vi "Main.vi"(11 "Module Admin":refnum<class "Delacor_lib_QMH_Module Admin.lvclass">) -> ()   [LabVIEW 2021, in "Main HMI.lvlib"]
doc: "This template is based off of the Queued Message Handler design pattern and the Queued Message Handler project template that ships with LabVIEW.\n\nThe main difference is that the queue is private to this module and communication between modules is performed via Broadcast and Request events.\n\nRequest events are wrapped in public API methods and are handled in the Event Handling Loop (EHL) of this VI. Any module can register for Broadcast events sent by this module. The EHL generates messages based on user interface actions.\n\nThe Message Handling Loop (MHL) processes messages generated by the EHL, or by other messages. The messages are string values, so new messages can be added easily to the Message Cases case structure in the MHL. Each message cluster can also provide an optional value for Message Data, which is a variant that can be converted to whatever message-specific data is required.\n_____\nBased on DQMH Dev Tools: Project Template 7.1.2.1547."
uses:
  Main HMI.lvlib
  <vilib>/Delacor/Delacor QMH/Libraries/Module Admin_class/Delacor_lib_QMH_Module Admin.lvclass
  Module Data--cluster.ctl
  Get Measurement from UDP HL--cluster.ctl
  Stop Argument--cluster.ctl
  <vilib>/Delacor/Delacor QMH/Libraries/Message Queue_class/Delacor_lib_QMH_Message Queue.lvclass/Delacor_lib_QMH_Message Queue.ctl
  <vilib>/Delacor/Delacor QMH/Libraries/Module Admin_class/Delacor_lib_QMH_Module Admin.lvclass/Delacor_lib_QMH_Module Admin.ctl
  Open UDP Connection Argument--cluster.ctl
  <vilib>/Utility/miscctls.llb/LVPointTypeDef.ctl
  <vilib>/Delacor/Delacor QMH/Libraries/Message Queue_class/Delacor_lib_QMH_Enqueue Message (Single).vi
  <vilib>/Delacor/Delacor QMH/Libraries/Module Admin_class/Delacor_lib_QMH_Get External Launch.vi
  <vilib>/Delacor/Delacor QMH/Libraries/Message Queue_class/Delacor_lib_QMH_Message Queue.lvclass
  Host Interpreter/Host Interpreter.lvlib
panel:
  out "Connected":bool
  in  "Disconnect from Target":bool
  in  "Connect to Target":bool
  out "CPU 2 (%)":u8(slide) scale=0.0..100.0
  out "CPU 1 (%)":u8(slide) scale=0.0..100.0
  out "Memory ROM Available (%)":u8(slide) scale=0.0..100.0
  out "Memory RAM Available (%)":u8(slide) scale=0.0..100.0
  out "Record Time":dbl format="%<%H:%M:%S%3u>t"
  in  "Record TDMS File":bool
  out "Analog Input":dbl[](array[numeric])
  out "Digital Input":bool[](array[boolean])
  out "error out":errorcluster
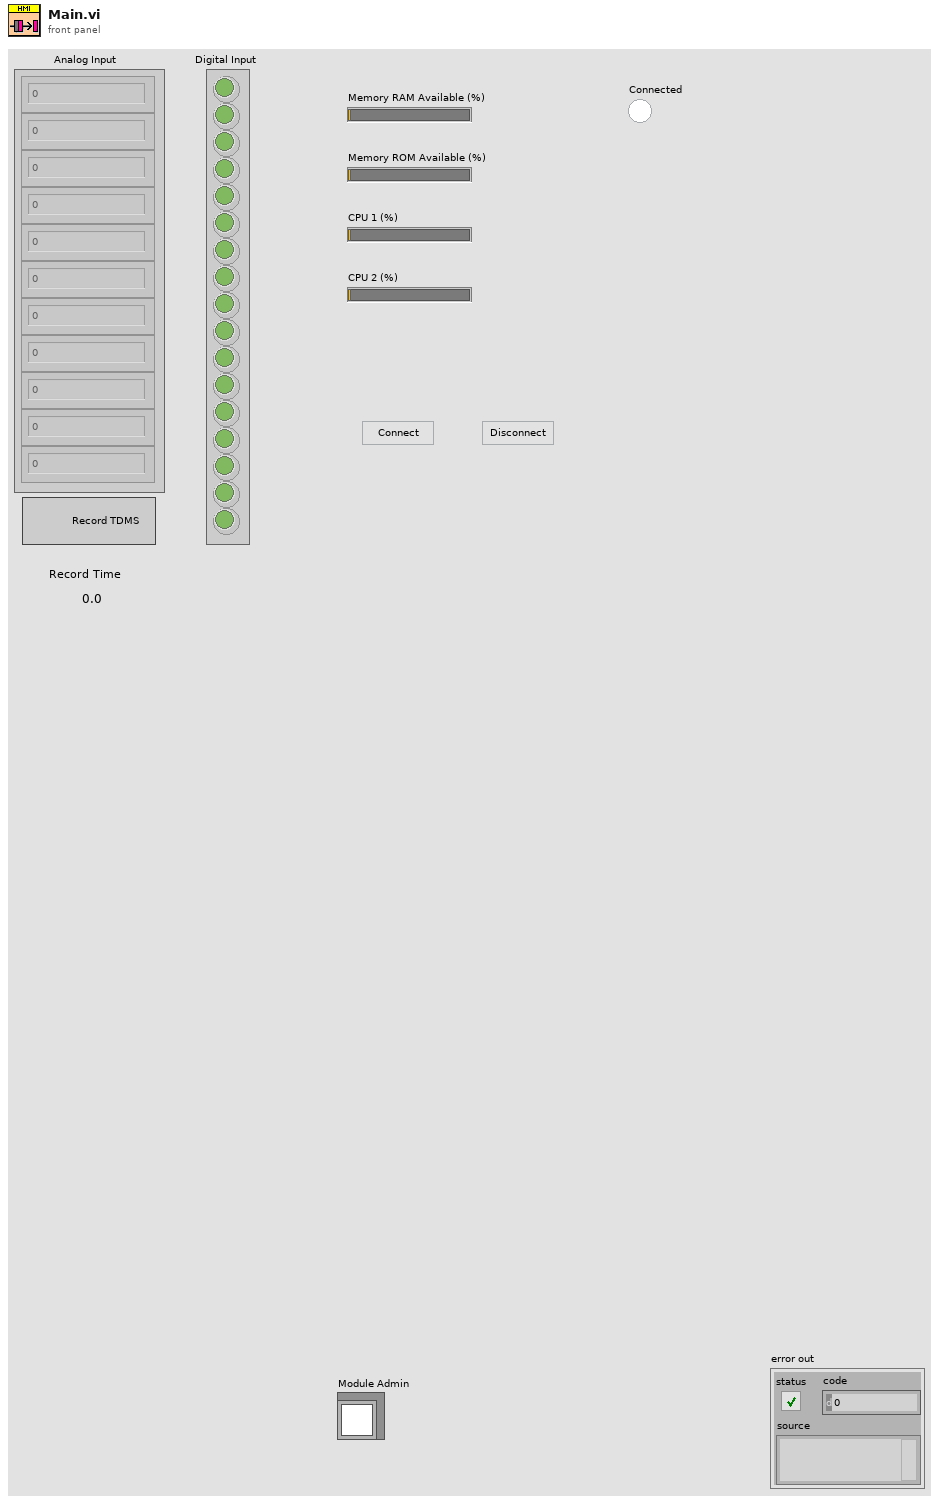
[diagram p1: front panel]
types:
  T1 = typedef "Main HMI.lvlib/Request Events--cluster.ctl" = cluster{"Stop Module":refnum<user-event>, "Show Panel":refnum<user-event>, "Hide Panel":refnum<user-event>, "Get Module Execution Status":refnum<user-event>, "Show Diagram":refnum<user-event>, "Private.Open UDP Connection":refnum<user-event>, "Private.Get UDP Info":refnum<user-event>, "Private.Recording":refnum<user-event>, "Update AIs":refnum<user-event>, "Update DOs Values":refnum<user-event>}
  T2 = typedef "Host Interpreter.lvlib/Broadcast Events--cluster.ctl" = cluster{"Module Did Init":refnum<user-event>, "Status Updated":refnum<user-event>, "Error Reported":refnum<user-event>, "Module Did Stop":refnum<user-event>, "Update Module Execution Status":refnum<user-event>, "Connected":refnum<user-event>, "Update Target Connections":refnum<user-event>, "Disconnected":refnum<user-event>}
  T3 = typedef "Main HMI.lvlib/Get Measurement from UDP HL--cluster.ctl" = cluster{"IP RT":string, "Port RT":u16, "Port Host":u16, "Recording?":bool, "Timestamp":timestamp}
  T4 = typedef "Main HMI.lvlib/Module Data--cluster.ctl" = cluster{"Status":string, "IP RT":string, "Port RT":u16, "Port Host":u16, "connection ID":refnum<k16>}
  T5 = enum32{"invalid lock state", "Not Locked", "Locked (No Password)", "Password-protected"}
  T6 = typedef "Main HMI.lvlib/Stop Argument--cluster.ctl" = cluster{"Origin":string, "Exit via Stop Module Req?":bool, "Wait for Module to stop?":bool}
  T7 = typedef "Main HMI.lvlib/Open UDP Connection Argument--cluster.ctl" = cluster{"Boolean":bool}
  T8 = typedef "LVPointTypeDef.ctl" = cluster{"Horizontal":i16, "Vertical":i16}
  T9 = enum32{"Invalid", "Standard", "Closed", "Hidden", "Minimized", "Maximized"}
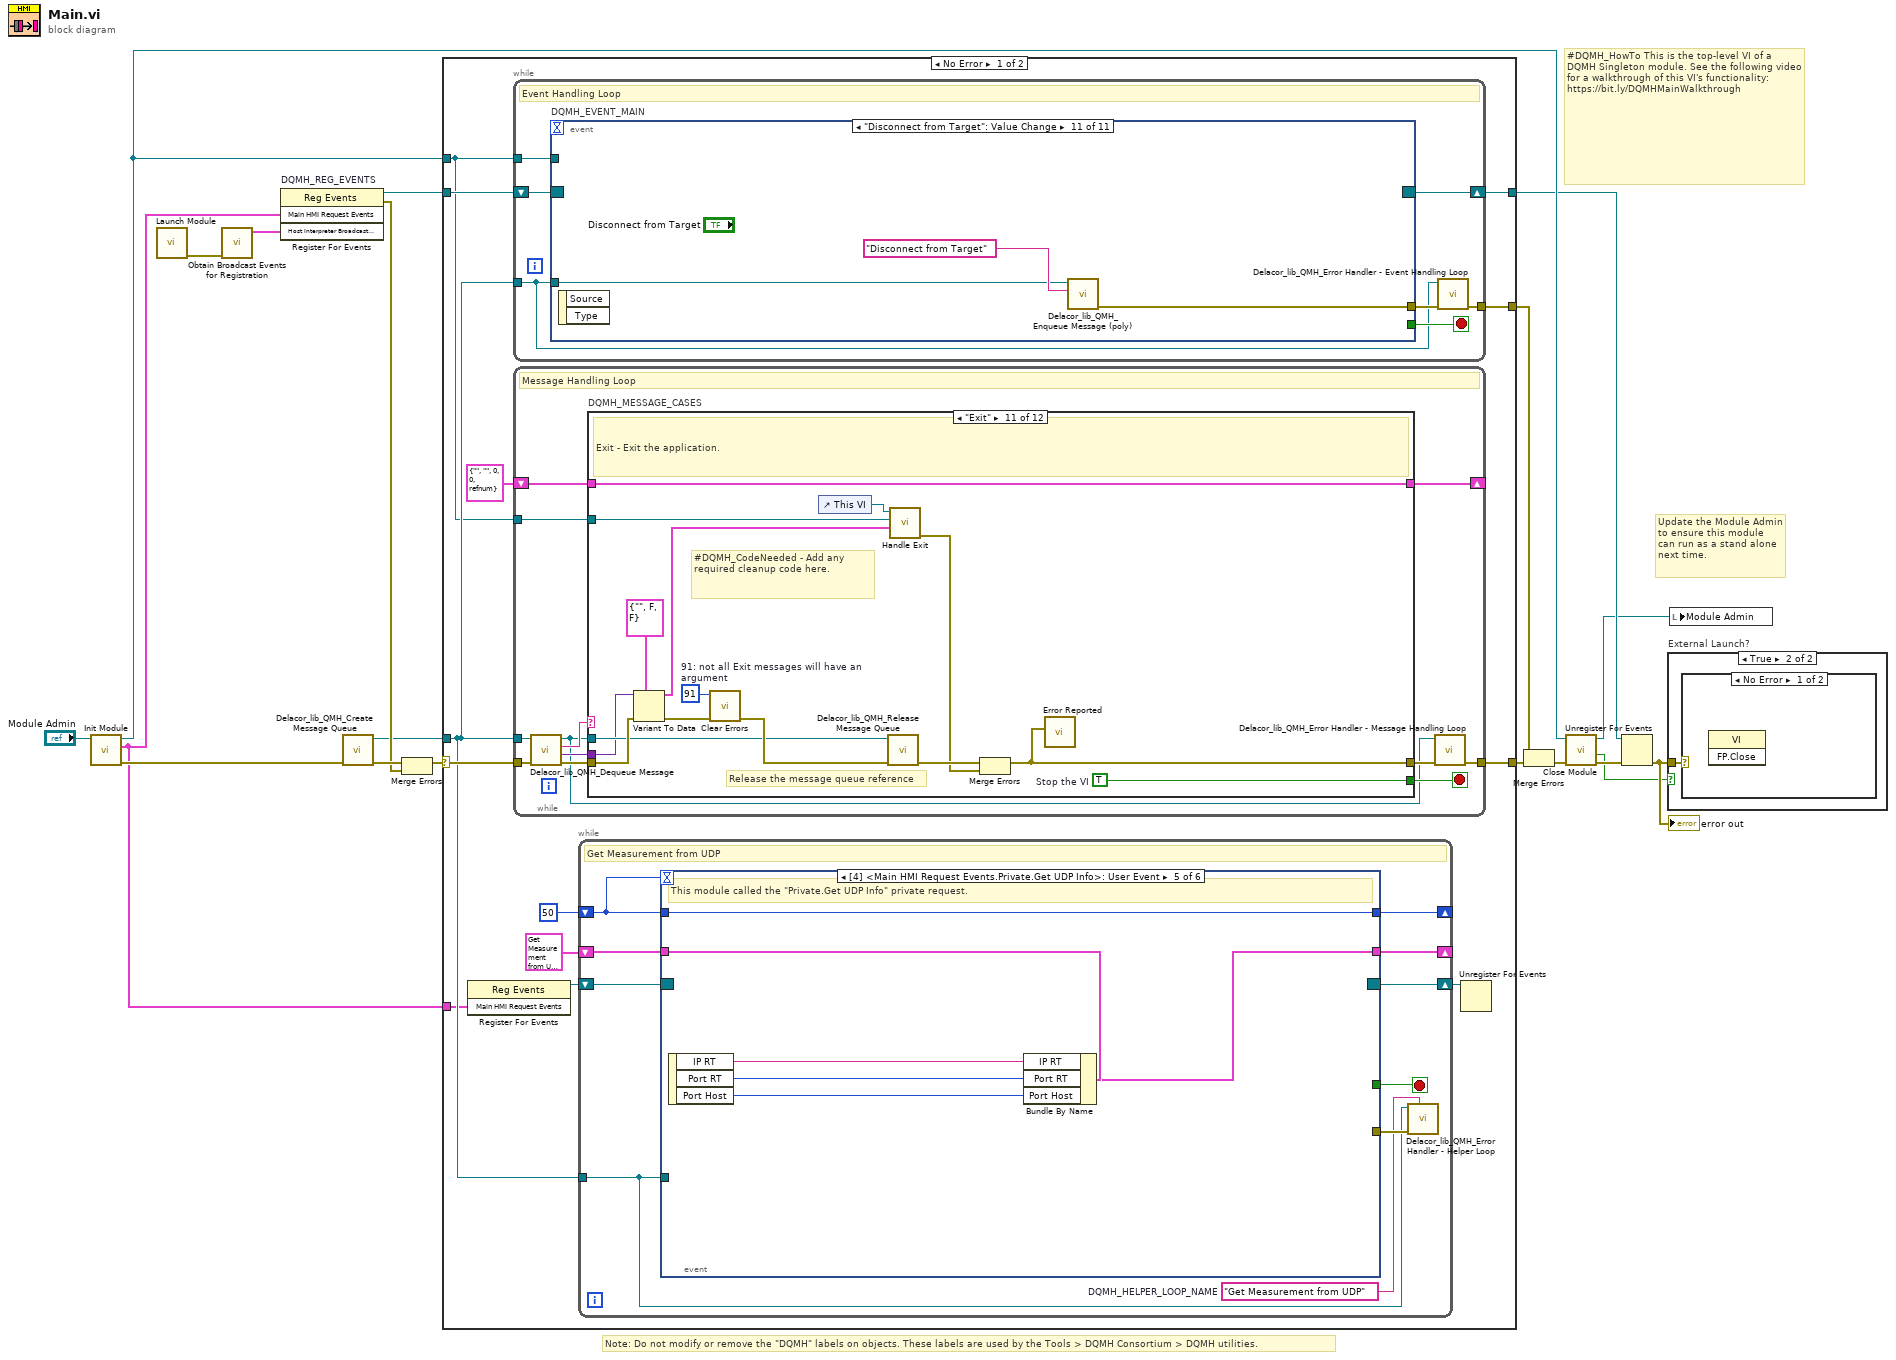
[diagram p0: block diagram]
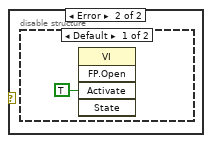
[diagram p3: hidden frame]
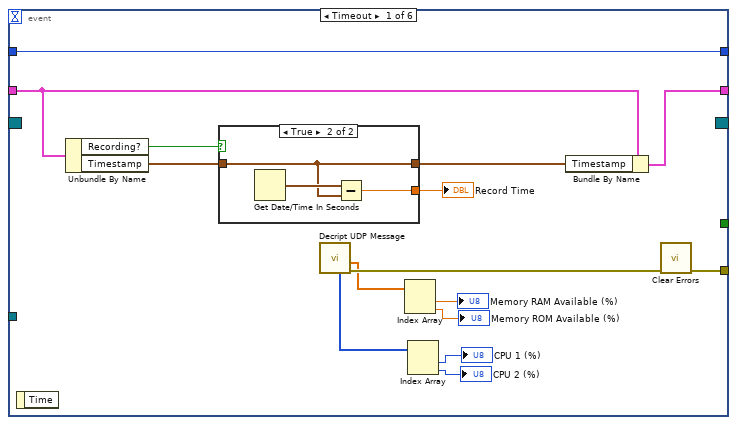
[diagram p5: hidden frame]
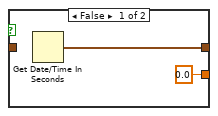
[diagram p6: hidden frame]
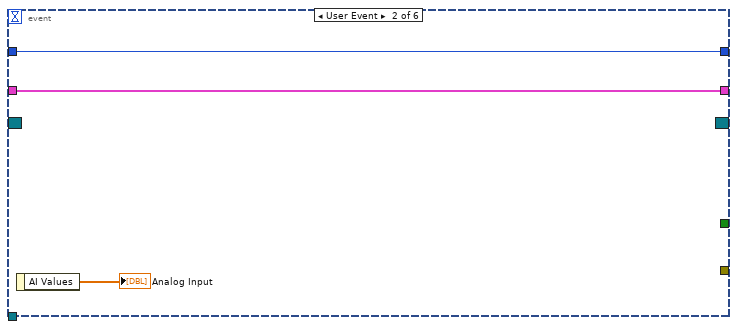
[diagram p7: hidden frame]
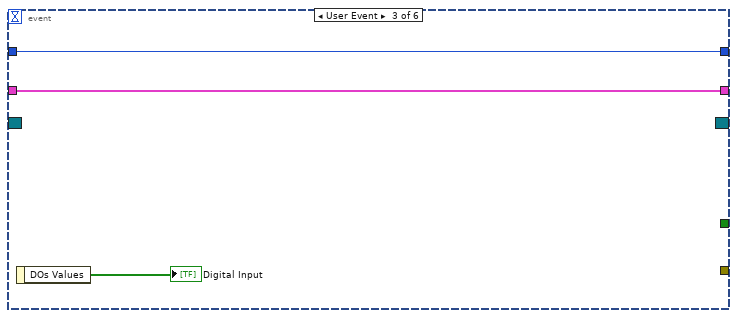
[diagram p8: hidden frame]
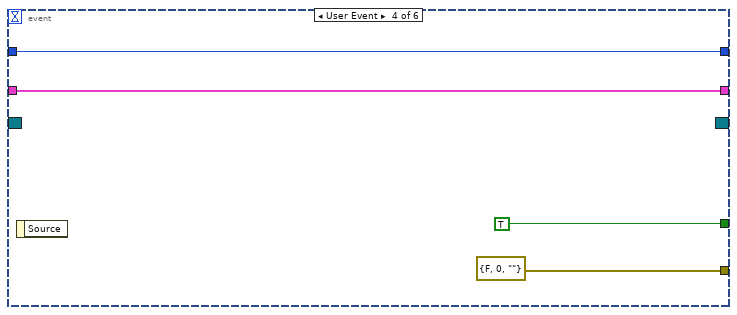
[diagram p9: hidden frame]
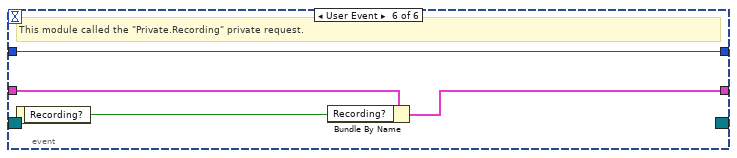
[diagram p10: hidden frame]
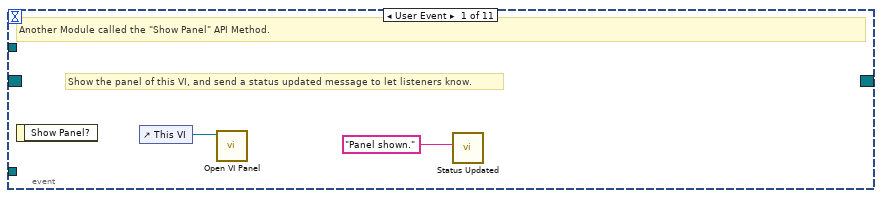
[diagram p11: hidden frame]
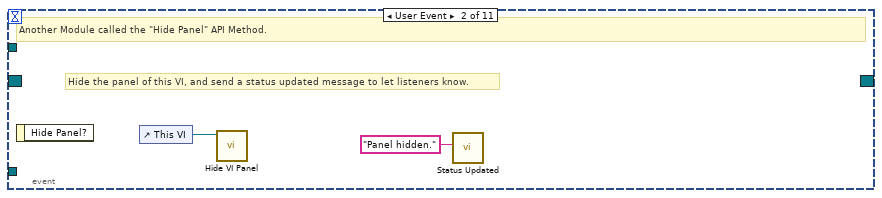
[diagram p12: hidden frame]
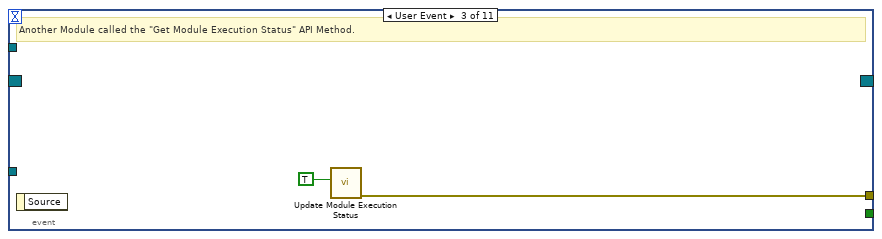
[diagram p13: hidden frame]
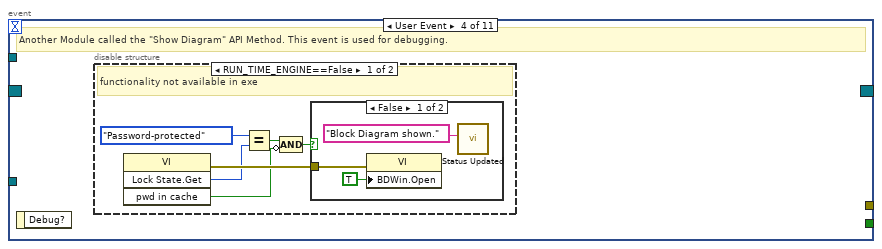
[diagram p14: hidden frame]
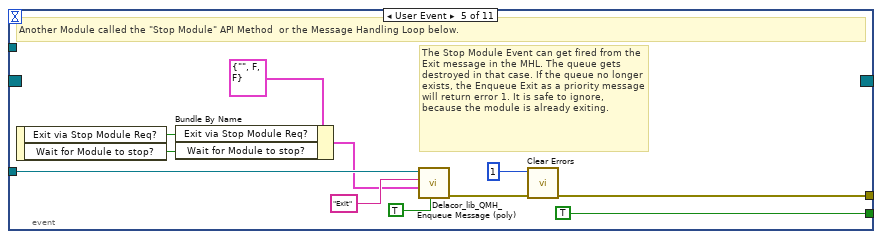
[diagram p17: hidden frame]
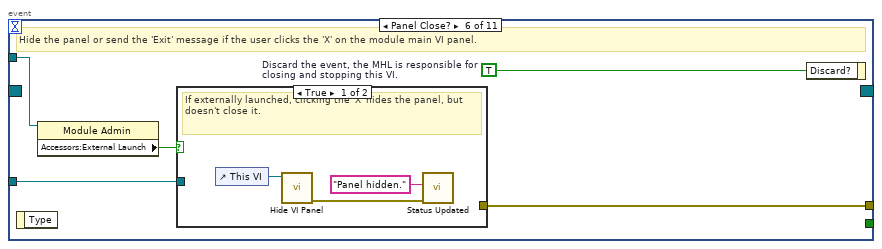
[diagram p18: hidden frame]
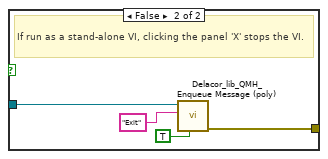
[diagram p19: hidden frame]
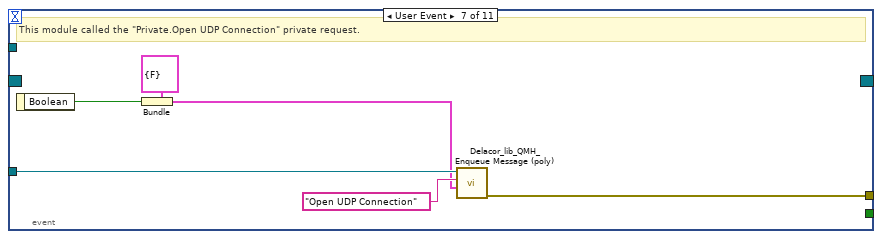
[diagram p20: hidden frame]
diagram:
  # "#DQMH_HowTo This is the top-level VI of a DQMH Singleton module. See the following video for a walkthrough of this VI's functionality: https://bit.ly/DQMHMainWalkthrough"
  # "Note: Do not modify or remove the \"DQMH\" labels on objects. These labels are used by the Tools > DQMH Consortium > DQMH utilities."
  # "Update the Module Admin to ensure this module can run as a stand alone next time."
  n1 = call "Init Module.vi"("Singleton Module Admin in"="Module Admin") -> ("error out"=w18:errorcluster, "Main HMI Request Events"=w3:T1, "Singleton Module Admin out"=w10:refnum<class "Delacor_lib_QMH_Module Admin.lvclass">)  [unwired: 8 in]
  n2 = call "Launch Module.vi"() -> ("error out"=w2:errorcluster)  [unwired: 11 in]
  n3 = call "Obtain Broadcast Events for Registration.vi"("error in"=w2) -> ("Host Interpreter Broadcast Events"=w1:T2)  [unwired: 8 in, 2 out]
  n4 = register-events "DQMH_REG_EVENTS"(w3, w1) -> (reference out=w8:refnum<event-registration>, error out=w11:errorcluster)  [unwired: 2 in]
  n5 = call <vilib>:"Delacor_lib_QMH_Create Message Queue.vi"("error in"=w18) -> ("error out"=w13:errorcluster, "Message Queue"=w7:refnum<class "Delacor_lib_QMH_Message Queue.lvclass">)  [unwired: 9 in]
  n6 = Merge Errors(w13, w11) -> (w12:errorcluster)
  n7 = case shown="No Error" w12 {
    selector: w12 -> [w30 w278]
    tunnel: [w32 w277] -> w19
    tunnel: [w29 w276] -> w9
    tunnel: w8 -> [w27 w276]
    tunnel: w7 -> [w26 w271]
    tunnel: [w31 _] -> w16
    tunnel: w10 -> [w25 w272]
    tunnel: w3 -> [w24 _]
    frame No Error {
      n8 = register-events ("DQMH_HELPER_REGFOREVENTS")(w24) -> (reference out=w22:refnum<event-registration>)  [unwired: 2 in, 1 out]
      n9 = while {
        tunnel: w26 -> [w83]
        shift-right: [w86] -> w29
        shift-left: w27 -> [w87]
        tunnel: [w88] -> w31
        tunnel: w25 -> [w84]
        stop <- w85 stop-if-true
        # "Event Handling Loop"
        n10 = event "DQMH_EVENT_MAIN" shown="[10] \"Disconnect from Target\": Value Change" {
          selector: w87 -> [_ _ _ _ _ _ _ _ _ _ _]
          dyn-events: [_ _ _ _ _ _ _ _ _ _ _] -> w86
          timeout: _ -> [_ _ _ _ _ _ _ _ _ _ _]
          tunnel: [_ _ _ _ TRUE ("Discard?") _ _ _ _ _ _] -> w85
          tunnel: w83 -> [_ _ _ _ w111 w118 w133 w137 w139 w142 w145]
          tunnel: [_ _ w95 _ w114 w120 w128 w135 w138 _ w144] -> w89
          tunnel: w84 -> [_ _ _ _ _ w117 _ _ _ _ _]
          event User Event {
            # "Show the panel of this VI, and send a status updated message to let listeners know."
            # "Another Module called the \"Show Panel\" API Method."
            n11 = event-data() -> ()  [unwired: 1 in, 1 out]
            n12 = control-ref of="This VI"() -> (w91:refnum<vi>)
            n13 = call "Open VI Panel.vi"("VI"=w91) -> ()  [unwired: 10 in, 1 out]
            n14 = call "Status Updated.vi"("Status"="Panel shown." ("format string")) -> ()  [unwired: 10 in, 1 out]
          }
          event User Event {
            # "Hide the panel of this VI, and send a status updated message to let listeners know."
            # "Another Module called the \"Hide Panel\" API Method."
            n15 = event-data() -> ()  [unwired: 1 in, 1 out]
            n16 = control-ref of="This VI"() -> (w93:refnum<vi>)
            n17 = call "Hide VI Panel.vi"("VI"=w93) -> ()  [unwired: 10 in, 1 out]
            n18 = call "Status Updated.vi"("Status"="Panel hidden." ("format string")) -> ()  [unwired: 10 in, 1 out]
          }
          event User Event {
            # "Another Module called the \"Get Module Execution Status\" API Method."
            n19 = event-data() -> ()  [unwired: 1 in, 1 out]
            n20 = call "Update Module Execution Status.vi"("Running?"=TRUE) -> ("error out"=w95:errorcluster)  [unwired: 10 in]
          }
          event User Event {
            # "Another Module called the \"Show Diagram\" API Method. This event is used for debugging."
            n21 = event-data() -> ()  [unwired: 1 in, 1 out]
            n22 = disable-structure shown="RUN_TIME_ENGINE==False" {
              frame condition #0 (active) {
                # "functionality not available in exe"
                n23 = invoke on="Invoke Node" class="VI" method="Lock State.Get"() -> (error out=w101:errorcluster, "Get Lock State"=w100:T5, "pwd in cache"=w97:bool)  [unwired: 4 in, 1 out]
                n24 = Equal?(x=T5."Password-protected", y=w100) -> (x = y?=w98:bool)
                n25 = Compound Arithmetic op=AND(w98, invert w97) -> (w96:bool)
                n26 = case shown="False" w96 {
                  tunnel: w101 -> [w104 _]
                  frame False {
                    n27 = property on="Property Node" class="VI"(error in=w104, "BDWin.Open"=TRUE ("Block Diagram Window:Open")) -> ()  [unwired: 1 in, 2 out]
                    n28 = call "Status Updated.vi"("Status"="Block Diagram shown." ("format string")) -> ()  [unwired: 10 in, 1 out]
                  }
                  frame True {
                    # "Password-protected VI, and the password is not in the cache. Do not show the diagram."
                  }
                }
              }
              frame condition #1 {
              }
            }
          }
          event User Event {
            # "The Stop Module Event can get fired from the Exit message in the MHL. The queue gets destroyed in that case. If the queue no longer exists, the Enqueue Exit as a priority message will return error 1. It is safe to ignore, because the module is already exiting."
            # "Another Module called the \"Stop Module\" API Method  or the Message Handling Loop below."
            n29 = event-data() -> ("Exit via Stop Module Req?"=w107:bool, "Wait for Module to stop?"=w106:bool)  [unwired: 1 in]
            n30 = Bundle By Name(cluster=T6 {"Origin"="", "Exit via Stop Module Req?"=FALSE, "Wait for Module to stop?"=FALSE} ("Stop Argument"), "Exit via Stop Module Req?"=w107, "Wait for Module to stop?"=w106) -> (w105:T6)
            n31 = call-poly <vilib>:"Delacor_lib_QMH_Enqueue Message (poly).vi"("Priority Message? (F)"=TRUE, "Message Data"=w105, "Message"="Exit", "Message Queue in"=w111) -> ("error out"=w115:errorcluster)  [unwired: 6 in, 1 out]
            n32 = call <vilib>:"Clear Errors.vi"("error in (no error)"=w115, "specific error code to clear (0: all)"=1) -> ("error out"=w114:errorcluster)  [unwired: 4 in, 1 out]
          }
          event Panel Close? {
            w119 = TRUE  # Discard the event, the MHL is responsible for closing and stopping this VI.
            # "Hide the panel or send the 'Exit' message if the user clicks the 'X' on the module main VI panel."
            n33 = event-data() -> ()  [unwired: 1 in, 1 out]
            n34 = property on="Property Node" class="Module Admin"(reference=w117) -> ("Accessors:External Launch"=w116:bool)  [unwired: 1 in, 2 out]
            n35 = case shown="True" w116 {
              tunnel: w118 -> [_ w126]
              tunnel: [_ w127] -> w120
              frame True {
                # "If externally launched, clicking the 'X' hides the panel, but doesn't close it."
                n36 = control-ref of="This VI"() -> (w123:refnum<vi>)
                n37 = call "Hide VI Panel.vi"("VI"=w123) -> ("error out"=w121:errorcluster)  [unwired: 10 in]
                n38 = call "Status Updated.vi"("error in"=w121, "Status"="Panel hidden." ("format string")) -> ()  [unwired: 9 in, 1 out]
              }
              frame False {
                # "If run as a stand-alone VI, clicking the panel 'X' stops the VI."
                n39 = call-poly <vilib>:"Delacor_lib_QMH_Enqueue Message (poly).vi"("Priority Message? (F)"=TRUE, "Message"="Exit", "Message Queue in"=w126) -> ("error out"=w127:errorcluster)  [unwired: 7 in, 1 out]
              }
            }
            n40 = event-data ("Event Filter Node")("Discard?"=w119) -> ()  [unwired: 1 in, 1 out]
          }
          event User Event {
            # "This module called the \"Private.Open UDP Connection\" private request."
            n41 = event-data() -> ("Boolean"=w129:bool)  [unwired: 1 in]
            n42 = Bundle(cluster=T7 {"Boolean"=FALSE} ("Open UDP Connection Argument"), "Boolean"=w129) -> (w130:T7)
            n43 = call-poly <vilib>:"Delacor_lib_QMH_Enqueue Message (poly).vi"("Message Data"=w130, "Message"="Open UDP Connection", "Message Queue in"=w133) -> ("error out"=w128:errorcluster)  [unwired: 7 in, 1 out]
          }
          event "Record TDMS File": Value Change {
            # "This module called the \"Private.Open UDP Connection\" private request."
            n44 = event-data() -> ("NewVal"=w134:bool)  [unwired: 1 in]
            n45 = call-poly <vilib>:"Delacor_lib_QMH_Enqueue Message (poly).vi"("Message Data"=w134, "Message"="Write UDP", "Message Queue in"=w137) -> ("error out"=w135:errorcluster)  [unwired: 7 in, 1 out]
          }
          event "Connect to Target": Value Change {
            n46 = event-data() -> ()  [unwired: 1 in, 2 out]
            n47 = call-poly <vilib>:"Delacor_lib_QMH_Enqueue Message (poly).vi"("Message"="Connect to Target", "Message Queue in"=w139) -> ("error out"=w138:errorcluster)  [unwired: 8 in, 1 out]
          }
          event User Event {
            n48 = event-data() -> ("Boolean"=w141:bool)  [unwired: 1 in]
            n49 = call-poly <vilib>:"Delacor_lib_QMH_Enqueue Message (poly).vi"("Message Data"=w141, "Message"="Connection Status Updated", "Message Queue in"=w142) -> ()  [unwired: 7 in, 2 out]
          }
          event "Disconnect from Target": Value Change {
            n50 = event-data() -> ()  [unwired: 1 in, 2 out]
            n51 = call-poly <vilib>:"Delacor_lib_QMH_Enqueue Message (poly).vi"("Message"="Disconnect from Target", "Message Queue in"=w145) -> ("error out"=w144:errorcluster)  [unwired: 8 in, 1 out]
          }
        }
        n52 = call-dynamic "Delacor_lib_QMH_Error Handler - Event Handling Loop.vi"("error in"=w89, "Message Queue in"=w83) -> ("dup error in"=w88:errorcluster)  [unwired: 8 in, 1 out]
      }
      n53 = while {
        tunnel: w26 -> [w147]
        shift-right: [w155] -> _
        shift-left: T4 {"Status"="", "IP RT"="", "Port RT"=0, "Port Host"=0, "connection ID"=refnum} ("Data Cluster") -> [w156]
        tunnel: w30 -> [w158]
        tunnel: [w150] -> w32
        tunnel: w25 -> [w151]
        stop <- w154 stop-if-true
        # "Message Handling Loop"
        n54 = call-dynamic "Delacor_lib_QMH_Dequeue Message.vi"("error in"=w158, "Message Queue in"=w147) -> ("error out"=w157:errorcluster, "Message Data"=w152:variant, "Message"=w153:string, "Message Queue out"=w148:refnum<class "Delacor_lib_QMH_Message Queue.lvclass">)  [unwired: 6 in]
        n55 = case "DQMH_MESSAGE_CASES" shown="\"Exit\"" w153 {
          selector: w153 -> [_ _ _ _ _ _ _ _ _ _ _ w266]
          tunnel: w148 -> [_ _ _ _ _ _ _ _ _ w232 w254 _]
          tunnel: w157 -> [w179 w183 w196 w211 w214 w216 w223 w226 w228 w239 w260 w269]
          tunnel: [w164 w183 w188 w198 w212 w215 w221 w225 w228 w235 w255 w270] -> w149
          tunnel: w156 -> [w162 w182 w193 w210 w213 w217 w222 w224 w227 w234 w253 w267]
          tunnel: [w163 w182 w194 w210 w213 w217 w222 w224 w227 w234 w253 w267] -> w155
          tunnel: [_ _ _ _ _ _ _ _ _ _ w252 _] -> w154
          tunnel: w152 -> [_ _ _ w206 _ _ w220 _ _ w233 w251 _]
          tunnel: w151 -> [w170 _ _ _ _ _ _ _ _ w231 w246 _]
          frame "Initialize" {
            # "Initialize - Any operation that needs to be done before the module can receive messages. Synchronize Caller Events.vi will inform Start Module.vi that the module has launched and is ready to receive messages. Module Did Init.vi will broadcast that the module initialized."
            n56 = call "Synchronize Caller Events.vi"("error in"=w179, "Singleton Module Admin in"=w170) -> ("error out"=w178:errorcluster, "Singleton Module Admin out"=w167:refnum<class "Delacor_lib_QMH_Module Admin.lvclass">)  [unwired: 8 in]
            n57 = property on="Property Node" class="Module Admin"(reference=w167) -> ("Accessors:External Launch"=w174:bool)  [unwired: 1 in, 2 out]
            n58 = Select(t=T9."Hidden" ("State"), s=w174, f=T9."Standard" ("State")) -> (s? t:f=w171:T9)
            n59 = call "Module Name--constant.vi"() -> ("Module Name"=w168:string)  [unwired: 11 in]
            n60 = call "Module Name--constant.vi"() -> ("Module Name"=w177:string)  [unwired: 11 in]
            n61 = property on="Property Node" class="VI"("Front Panel.Title"=w177) -> (reference out=w176:refnum<vi>, error out=w181:errorcluster)  [unwired: 2 in]
            n62 = Bundle By Name(cluster=w162, "IP RT"="192.168.1.163", "Port RT"=u16 61670, "Port Host"=u16 12390) -> (w163:T4)
            n63 = call "Module Did Init.vi"("error in"=w178, "Initialized?"=TRUE, "Origin"=w168) -> ("error out"=w165:errorcluster)  [unwired: 8 in]
            n64 = invoke on="Invoke Node" class="VI" method="FP.Open"(reference=w176, error in=w181, "State"=w171) -> (reference out=w175:refnum<vi>, error out=w180:errorcluster)  [unwired: 2 in, 3 out]
            n65 = invoke on="Invoke Node" class="VI" method="FP.Center"(reference=w175, error in=w180) -> ()  [unwired: 1 in, 3 out]
            n66 = property on="Pane" class="Pane"("Origin"=T8 {"Horizontal"=0, "Vertical"=0}) -> ()  [unwired: 2 in, 2 out]
            n67 = call "Open UDP Connection.vi"("error in"=w165) -> ("error out"=w164:errorcluster)  [unwired: 10 in]
          }
          frame "---Module Specific---" {
            # "Separator -- The following cases handle messages specific to this Module."
          }
          frame "Open UDP Connection" {
            # "Open UDP Connection"
            n68 = Unbundle By Name(w193) -> ("Port RT"=w184:u16, "IP RT"=w185:string, "Port Host"=w186:u16)
            n69 = String To IP(1:w185) -> (0:w190:u32)
            n70 = UDP Open(8:w196, 11:w186) -> (port=w192:refnum<k16>, 0:w195:errorcluster)  [unwired: 3 in, 1 out]
            n71 = UDP Write(address=w190, port or service name=w184, connection ID=w192, data in="start", 8:w195) -> (error out=w189:errorcluster, 3:w187:refnum<k16>)  [unwired: 1 in]
            n72 = Bundle By Name(cluster=w193, "connection ID"=w187) -> (w194:T4)
            n73 = call "Get UDP Info.vi"("connection ID"=w187, "Port Host"=w186, "error in"=w189, "Port RT"=w184, "IP RT"=w185) -> ("error out"=w188:errorcluster)  [unwired: 6 in]
          }
          frame "Write UDP" {
            # "Write UDP"
            n74 = Variant To Data(error in=w211, type=FALSE, Variant=w206) -> (data=w197:bool, error out=w208:errorcluster)
            n75 = Type Cast(type=u8[] [], x=w197) -> (*(type *) &x=w204:u8[])
            n76 = Byte Array To String(unsigned byte array=w204) -> (string=w203:string)
            n77 = Unbundle By Name(w210) -> ("Port RT"=w202:u16, "IP RT"=w201:string, "connection ID"=w209:refnum<k16>)
            n78 = String To IP(1:w201) -> (0:w200:u32)
            n79 = UDP Write(address=w200, port or service name=w202, connection ID=w209, data in=w203, 8:w208) -> (error out=w199:errorcluster)  [unwired: 1 in, 1 out]
            n80 = call "Recording.vi"("error in"=w199, "Recording?"=w197) -> ("error out"=w198:errorcluster)  [unwired: 9 in]
          }
          frame "Connect to Target" {
            n81 = call "Connect to Target.vi"("error in"=w214) -> ("error out"=w212:errorcluster)  [unwired: 10 in]
          }
          frame "Disconnect from Target" {
            n82 = call "Disconnect from Target.vi"("error in"=w216) -> ("error out"=w215:errorcluster)  [unwired: 10 in]
          }
          frame "Connection Status Updated" {
            n83 = Variant To Data(error in=w223, type=FALSE, Variant=w220) -> (data=→"Connected":bool, error out=w221:errorcluster)
          }
          frame "---Copy This Frame---" {
            # "Duplicate this frame when creating new messages.  Change this comment in the duplicated frame to describe this message."
            n84 = Merge Errors(w226) -> (w225:errorcluster)
          }
          frame "---Exit and Error Handling---" {
            # "Separator - The following cases handle errors and exit messages."
          }
          frame "Error" {
            # "#DQMH_CodeRecommended - If the module is running in standalone mode (External Launch = FALSE), this code will pop up an error dialog and call the 'Exit' message if an error occurs. Add more fine-grained error management here."
            # "Error - Check the error message data and respond accordingly. This message is sent by the \"Error Handler\" VIs at the end of each loop in this application."
            n85 = property on="Property Node" class="Module Admin"(reference=w231) -> ("Accessors:External Launch"=w230:bool)  [unwired: 1 in, 2 out]
            n86 = Variant To Data(error in=w239, type=errorcluster {"status"=FALSE, "code"=0, "source"=""} ("error constant"), Variant=w233) -> (data=w229:errorcluster, error out=w237:errorcluster)
            n87 = local write "error out"(w229) -> ()
            n88 = call "Error Reported.vi"("Error"=w229) -> ()  [unwired: 10 in, 1 out]
            n89 = case shown="False" w230 {
              tunnel: [w244 _] -> w236
              tunnel: w232 -> [w242 _]
              tunnel: w229 -> [w243 _]
              frame False {
                n90 = disable-structure shown="Default" {
                  disable-tunnel: w243 -> [w245 _]
                  frame condition #0 (active) {
                    # "If the module is running standalone, then pop up an error dialog and call the \"Exit\" message."
                    n91 = call <vilib>:"Simple Error Handler.vi"("error in (no error)"=w245) -> ()  [unwired: 4 in, 5 out]
                  }
                  frame condition #1 {
                    # "To prevent the Simple Error Handler VI from being loaded (e.g. when deploying to a Real-Time target), add the Conditional Disable Symbol \"DQMH_Disable_SEH\" to your project and set it to TRUE."
                  }
                }
                n92 = call-poly <vilib>:"Delacor_lib_QMH_Enqueue Message (poly).vi"("Priority Message? (F)"=TRUE, "Message"="Exit", "Message Queue in"=w242) -> ("error out"=w244:errorcluster)  [unwired: 7 in, 1 out]
              }
              frame True {
                # "If the module was launched externally, calling the Error Reported broadcast VI is the only action performed by the \"Error\" message. The module's caller can then process the error appropriately."
              }
            }
            n93 = Merge Errors(w237, w236) -> (w235:errorcluster)
          }
          frame "Exit" {
            w250 = 91  # 91: not all Exit messages will have an argument
            w252 = TRUE  # Stop the VI
            # "Release the message queue reference"
            # "#DQMH_CodeNeeded - Add any required cleanup code here."
            # "Exit - Exit the application."
            n94 = Variant To Data(error in=w260, type=T6 {"Origin"="", "Exit via Stop Module Req?"=FALSE, "Wait for Module to stop?"=FALSE} ("Stop Argument"), Variant=w251) -> (data=w248:T6, error out=w257:errorcluster)
            n95 = call <vilib>:"Clear Errors.vi"("error in (no error)"=w257, "specific error code to clear (0: all)"=w250) -> ("error out"=w259:errorcluster)  [unwired: 4 in, 1 out]
            n96 = control-ref of="This VI"() -> (w247:refnum<vi>)
            n97 = call-dynamic "Delacor_lib_QMH_Release Message Queue.vi"("error in"=w259, "Message Queue"=w254) -> ("error out"=w258:errorcluster)  [unwired: 9 in]
            n98 = call "Handle Exit.vi"("Stop Argument"=w248, "Admin in"=w246, "VI reference"=w247) -> ("error out"=w256:errorcluster)  [unwired: 7 in, 1 out]
            n99 = Merge Errors(w258, w256) -> (w255:errorcluster)
            n100 = call "Error Reported.vi"("Error"=w255) -> ()  [unwired: 10 in, 1 out]
          }
          frame Default {
            # "'Default' case only runs if there is a message that isn't defined in any of the other cases.  Output a programming error."
            n101 = call "Module Name--constant.vi"() -> ("Module Name"=w265:string)  [unwired: 11 in]
            n102 = Format Into String(format string="The invalid message string \"%s\" was received in the Message Handling Loop for module \"%s\".", w266, w265) -> (resulting string=w261:string)  [unwired: 2 in, 1 out]
            n103 = call <vilib>:"Error Cluster From Error Code.vi"("show call chain? (False)"=TRUE, "error message (\"\")"=w261, "error code (0)"=1) -> ("error out"=w268:errorcluster)  [unwired: 6 in]
            n104 = Merge Errors(w269, w268) -> (w270:errorcluster)
          }
        }
        n105 = call-dynamic "Delacor_lib_QMH_Error Handler - Message Handling Loop.vi"("error in"=w149, "Message Queue in"=w148) -> ("dup error in"=w150:errorcluster)  [unwired: 8 in, 1 out]
      }
      n106 = while "DQMH_HELPER_LOOP" {
        shift-right: [w42] -> _
        shift-left: 50 -> [w41]
        shift-right: [w39] -> w23
        shift-left: w22 -> [w40]
        tunnel: w26 -> [w36]
        shift-right: [w34] -> _
        shift-left: T3 {"IP RT"="", "Port RT"=0, "Port Host"=0, "Recording?"=FALSE, "Timestamp"=timestamp(0 s since 1904-01-01)} ("Get Measurement from UDP HL--cluster") -> [w33]
        stop <- w38 stop-if-true
        w35 = "Get Measurement from UDP"  # DQMH_HELPER_LOOP_NAME
        # "Get Measurement from UDP"
        n107 = event "DQMH_HELPER_EVENT_STRUCTURE" shown="[4] <Main HMI Request Events.Private.Get UDP Info>: User Event" {
          selector: w40 -> [_ _ _ _ _ _]
          dyn-events: [_ _ _ _ _ _] -> w39
          timeout: w41 -> [_ _ _ _ _ _]
          tunnel: w41 -> [w57 w65 w68 w72 w78 w82]
          tunnel: [w57 w65 w68 w72 w78 w82] -> w42
          tunnel: [_ _ _ TRUE _ _] -> w38
          tunnel: [w56 _ _ errorcluster {"status"=FALSE, "code"=0, "source"=""} ("error constant") _ _] -> w37
          tunnel: w36 -> [_ _ _ _ _ _]
          tunnel: [w44 w64 w67 w69 w73 w80] -> w34
          tunnel: w33 -> [w47 w64 w67 w69 w77 w81]
          event Timeout {
            n108 = event-data() -> ()  [unwired: 1 in, 1 out]
            n109 = Unbundle By Name(w47) -> ("Recording?"=w46:bool, "Timestamp"=w45:timestamp)
            n110 = case shown="True" w46 {
              tunnel: [w59 w61] -> w43
              tunnel: w45 -> [_ w61]
              tunnel: [0.0 w60] -> w54
              frame False {
                n111 = Get Date/Time In Seconds() -> (seconds since 1Jan1904=w59:timestamp)
              }
              frame True {
                n112 = Get Date/Time In Seconds() -> (seconds since 1Jan1904=w62:timestamp)
                n113 = Subtract(x=w62, y=w61) -> (x-y=w60:dbl)
              }
            }
            "Record Time" <- w54
            n114 = call "Decript UDP Message.vi"() -> ("Error Out"=w55:errorcluster, "Memory"=w53:dbl[], "CPU"=w50:u32[])  [unwired: 7 in, 2 out]
            n115 = Index Array(array=w53) -> (element #1=→"Memory RAM Available (%)":dbl, element #2=→"Memory ROM Available (%)":dbl)  [unwired: 2 in]
            n116 = Index Array(array=w50) -> (element #1=→"CPU 1 (%)":u32, element #2=→"CPU 2 (%)":u32)  [unwired: 2 in]
            n117 = Bundle By Name(cluster=w47, "Timestamp"=w43) -> (w44:T3)
            n118 = call <vilib>:"Clear Errors.vi"("error in (no error)"=w55) -> ("error out"=w56:errorcluster)  [unwired: 5 in, 1 out]
          }
          event User Event {
            n119 = event-data() -> ("AI Values"=→"Analog Input":sgl[])  [unwired: 1 in]
          }
          event User Event {
            n120 = event-data() -> ("DOs Values"=→"Digital Input":bool[])  [unwired: 1 in]
          }
          event User Event {
            n121 = event-data() -> ()  [unwired: 1 in, 1 out]
          }
          event User Event {
            # "This module called the \"Private.Get UDP Info\" private request."
            n122 = event-data() -> ("IP RT"=w76:string, "Port RT"=w75:u16, "Port Host"=w74:u16)  [unwired: 1 in]
            n123 = Bundle By Name(cluster=w77, "IP RT"=w76, "Port RT"=w75, "Port Host"=w74) -> (w73:T3)
          }
          event User Event {
            # "This module called the \"Private.Recording\" private request."
            n124 = event-data() -> ("Recording?"=w79:bool)  [unwired: 1 in]
            n125 = Bundle By Name(cluster=w81, "Recording?"=w79) -> (w80:T3)
          }
        }
        n126 = call-dynamic "Delacor_lib_QMH_Error Handler - Helper Loop.vi"("Error Debug"=w35, "error in"=w37, "Message Queue in"=w36) -> ()  [unwired: 7 in, 2 out]
      }
      n127 = Unregister For Events(event registration refnum=w23) -> ()  [unwired: 1 in, 1 out]
    }
    frame Error {
      # "Synchronize Caller Events.vi will inform Start Module.vi that the module has launched and will let the code calling Start Module.vi register for broadcasts and would permit the caller receive the broadcast that an error occurred at launch time."
      n128 = call-dynamic "Delacor_lib_QMH_Release Message Queue.vi"("error in"=w278, "Message Queue"=w271) -> ("error out"=w277:errorcluster)  [unwired: 9 in]
      n129 = call "Synchronize Caller Events.vi"("Singleton Module Admin in"=w272) -> ("error out"=w279:errorcluster)  [unwired: 9 in, 1 out]
      n130 = call "Module Name--constant.vi"() -> ("Module Name"=w275:string)  [unwired: 11 in]
      n131 = Format Into String(format string="An error occurred during initialization. %s is no longer running.", w275) -> (resulting string=w273:string)  [unwired: 2 in, 1 out]
      n132 = Merge Errors(w277, w279) -> (w280:errorcluster)
      n133 = call "Error Reported.vi"("Additional Information"=w273, "Error"=w280) -> ()  [unwired: 9 in, 1 out]
    }
  }
  n134 = Merge Errors(w16, w19) -> (w15:errorcluster)
  n135 = call "Close Module.vi"("error in"=w15, "Module Admin in"=w10) -> ("error out"=w17:errorcluster, "External Launch"=w4:bool, "Module Admin out"=w5:refnum<class "Delacor_lib_QMH_Module Admin.lvclass">)  [unwired: 7 in]
  n136 = Unregister For Events(event registration refnum=w9, error in=w17) -> (error out=w14:errorcluster)
  "error out" <- w14
  n137 = case "External Launch?" shown="True" w4 {
    tunnel: w14 -> [_ w281]
    frame False {
    }
    frame True {
      n138 = case shown="No Error" w281 {
        frame No Error {
          n139 = invoke on="Invoke Node" class="VI" method="FP.Close"() -> ()  [unwired: 3 in, 3 out]
        }
        frame Error {
          n140 = disable-structure shown="Default" {
            frame condition #0 (active) {
              n141 = invoke class="VI" method="FP.Open"("Activate"=TRUE ("Activate?")) -> ()  [unwired: 4 in, 5 out]
            }
            frame condition #1 {
              # "Don't show panel on error if running inside a built EXE."
            }
          }
        }
      }
    }
  }
  n142 = local write "Module Admin"(w5) -> ()
